vi "Get Student Info.vi"(8 "Error In":errorcluster, 11 "Path In":path) -> (0 "Error Out":errorcluster, 1 "Student Info":T1, 2 "Found Usr Cfg File?":bool=TRUE, 3 "Path Out":path)   [LabVIEW 2014]
uses:
  Ctls/Student Info.ctl
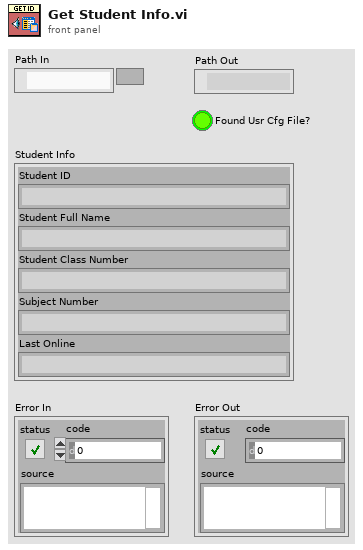
[diagram p1: front panel]
types:
  T1 = typedef "Student Info.ctl" = cluster{"Student ID":string, "Student Full Name":string, "Student Class Number":string, "Subject Number":string, "Last Online":string}
  T2 = enum16{"open", "replace", "create", "open or create", "replace or create", "replace or create with confirmation"}
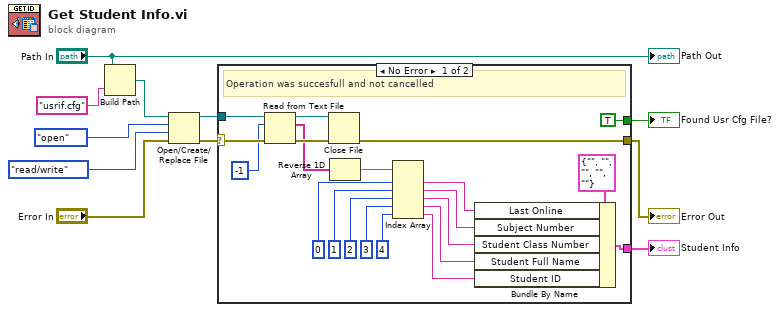
[diagram p0: block diagram]
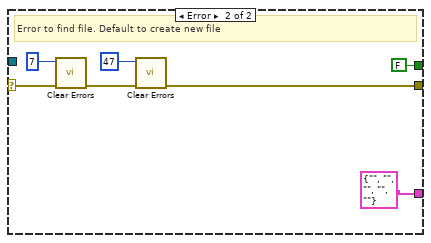
[diagram p2: hidden frame]
diagram:
  n1 = Build Path(base path="Path In", name or relative path="usrif.cfg") -> (appended path=w10:path)
  n2 = Open/Create/Replace File(file path (use dialog)=w10, error in="Error In", operation (0:open)=T2."open", access (0:read/write)=enum16{"read/write", "read-only", "write-only"}."read/write") -> (refnum out=w4:refnum<file>, error out=w5:errorcluster)  [unwired: 2 in, 1 out]
  n3 = case shown="No Error" w5 {
    selector: w5 -> [w31 w37]
    tunnel: w4 -> [w32 _]
    tunnel: [w14 T1 {"Student ID"="", "Student Full Name"="", "Student Class Number"="", "Subject Number"="", "Last Online"=""} ("Student Info")] -> w3
    tunnel: [w13 w35] -> w2
    tunnel: [TRUE FALSE] -> w1
    frame No Error {
      # "Operation was succesfull and not cancelled"
      n4 = Read from Text File(file (use dialog)=w32, count=-1, error in=w31) -> (refnum out=w30:refnum<file>, text=w27:string[], error out=w29:errorcluster)  [unwired: 1 in, 1 out]
      n5 = Close File(refnum=w30, error in=w29) -> (error out=w13:errorcluster)  [unwired: 1 out]
      n6 = Reverse 1D Array(array=w27) -> (reversed array=w26:string[])
      n7 = Index Array(array=w26, index #1=0 ("count"), index #2=1 ("count"), index #3=2 ("count"), index #4=3 ("count"), index #5=4 ("count")) -> (element #1=w19:string, element #2=w18:string, element #3=w17:string, element #4=w16:string, element #5=w15:string)
      n8 = Bundle By Name(cluster=T1 {"Student ID"="", "Student Full Name"="", "Student Class Number"="", "Subject Number"="", "Last Online"=""} ("Student Info"), "Last Online"=w19, "Subject Number"=w18, "Student Class Number"=w17, "Student Full Name"=w16, "Student ID"=w15) -> (w14:T1)
    }
    frame Error {
      # "Error to find file. Default to create new file"
      n9 = call <vilib>:"Clear Errors.vi"("error in (no error)"=w37, "specific error code to clear (0: all)"=7) -> ("error out"=w36:errorcluster)  [unwired: 4 in, 1 out]
      n10 = call <vilib>:"Clear Errors.vi"("error in (no error)"=w36, "specific error code to clear (0: all)"=47) -> ("error out"=w35:errorcluster)  [unwired: 4 in, 1 out]
    }
  }
  "Error Out" <- w2
  "Found Usr Cfg File?" <- w1
  "Student Info" <- w3
  "Path Out" <- "Path In"
